vi "Dashboard Main.vi"() -> ()   [LabVIEW 2020]
uses:
  <vilib>/Rock Robotics/WPI/Dashboard/WPI_DashboardLogging Global.vi
  <vilib>/Rock Robotics/Network Tables/NT Read Numeric Array.vi
  <vilib>/Analysis/NI_AALPro.lvlib
  <vilib>/Analysis/coordinate.llb/2D Cartesian Coordinate Rotation (Scalar).vi
  <vilib>/Analysis/NI_AAL_Angle.lvlib
  <vilib>/Analysis/coordinate.llb/Angle Units.ctl
  <vilib>/Analysis/coordinate.llb/Wrap Angle (scalar).vi
panel:
  out "NT Connection":bool
  in  "Camera Settings Right":T1={"Frame Rate"=30, "Compression"=30, "Size"=1, "DB Camera Config"=FALSE} {"Frame Rate" scale=1.0..30.0; "Compression" scale=100.0..-1.0; "Size" items=["640x480", "320x240", "160x120"]}
  in  "Camera Name Right":string(combo)="No Camera Selection"
  out "Camera Perf":string
  in  "Camera Settings":T1={"Frame Rate"=30, "Compression"=30, "Size"=1, "DB Camera Config"=FALSE} {"Frame Rate" scale=1.0..30.0; "Compression" scale=100.0..-1.0; "Size" items=["640x480", "320x240", "160x120"]}
  in  "TCP":refnum<k5>
  in  "Rec Mode":enum32{"Stop", "Record", "Playback"}(radio)
  out "Robot IP":string
  out "Image Message":string="Timeout in Camera Communications"
  in  "Dashboard Tab":T2(tab)
  out "Mode":T3(ring)=enum."Auto Disabled"
  out "Right Camera Perf":cluster{"Bandwidth (Mbps)":dbl, "FPS":dbl}
  out "Swerve Visualizer":cluster{dbl[], dbl[]}[](graph)
  out "Pod Comparisons (Diff -> Setpoint - Actual)":T4
  out "Pose":cluster{"x":dbl, "y":dbl, "theta":dbl}
  out "?":picture
  out "RR":bool=TRUE
  out "Velocity Setpoint":cluster{"vx":dbl, "vy":dbl, "w":dbl}
  out "Estimated Velocity":cluster{"vx":dbl, "vy":dbl, "w":dbl}
  out "Camera Image Right":T5(plugin-control)
  in  "Test Slider":dbl(slide) scale=0.0..100.0 scale format="%#_3g"
  in  "On/Off":bool caption="Solenoid"
  in  "Test Name":u16(ring) items=["Select the test to run..."]
  in  "Test Tree":string(tree)
  in  "Motor":cluster{"Value":dbl, "Enable":bool} {"Value" scale=-1.0..1.0 scale format="%#_3g"}
  out "Progress":T6 {"Test Progress" scale=0.0..100.0}
  in  "Rev/Fwd":cluster{"Forward":bool, "Reverse":bool}
  in  "Test Ring":u16(ring) items=["Monochrome", "Color"]
  out "Tree":string(tree)
  out "Camera Image":T5(plugin-control)
  out "Background":bool
  in  "Camera Name":string(combo)="No Camera Selection"
  # "HW"
  # "HW"
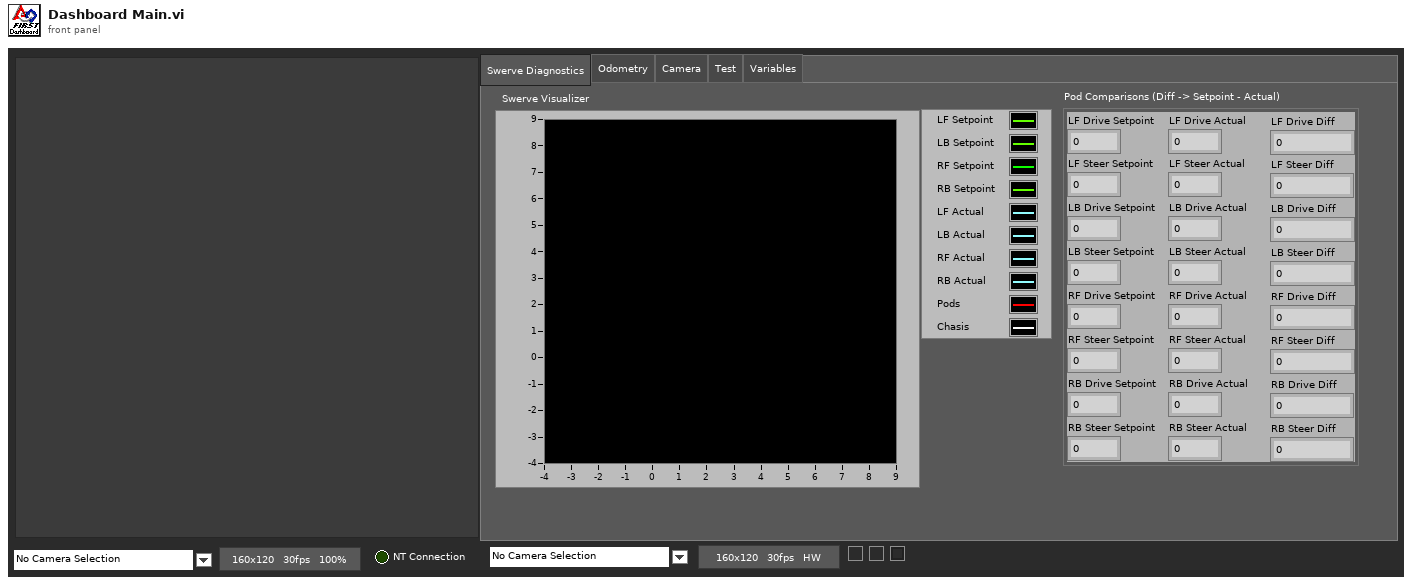
[diagram p1: front panel]
types:
  T1 = cluster{"Frame Rate":i32, "Compression":i32, "Size":u16, "DB Camera Config":bool}
  T2 = enum32{"Swerve Diagnostics", "Odometry", "Camera", "Test", "Variables"}
  T3 = enum8{"Tele-Op Disabled", "Tele-Op Enabled", "Auto Disabled", "Auto Enabled", "Test Disabled", "Test Enabled", "Disconnected", "No Code", "E-Stop"}
  T4 = cluster{"LF Drive Setpoint":dbl, "LF Steer Setpoint":dbl, "LB Drive Setpoint":dbl, "LB Steer Setpoint":dbl, "RF Drive Setpoint":dbl, "RF Steer Setpoint":dbl, "RB Drive Setpoint":dbl, "RB Steer Setpoint":dbl, "LF Drive Actual":dbl, "LF Steer Actual":dbl, "LB Drive Actual":dbl, "LB Steer Actual":dbl, "RF Drive Actual":dbl, "RF Steer Actual":dbl, "RB Drive Actual":dbl, "RB Steer Actual":dbl, "LF Drive Diff":dbl, "LF Steer Diff":dbl, "LB Drive Diff":dbl, "LB Steer Diff":dbl, "RF Drive Diff":dbl, "RF Steer Diff":dbl, "RB Drive Diff":dbl, "RB Steer Diff":dbl}
  T5 = typedef "IMAQ Image.ctl" = refnum<image>
  T6 = cluster{"Test Progress":u8, "Test Progress Text":string}
  T7 = cluster{"Save Path":path, "Interval (s)":dbl, "Keep":i32}
  T8 = typedef "Image Type" = u32
  T9 = cluster{"Error Strings":string, "Disable Counts":cluster{u16, u16}, "Rail Faults":cluster{u16, u16, u16}, "Robot IP":string, "DB Mode":u8, "Event Info":cluster{"Name":string, "Type":u8, "Number":u16, "Replay":u8}}
  T10 = cluster{"Storage":cluster{"Disk Free":u64, "RAM Block":u32, "RAM free":u32}, "CPU Utilization":cluster{"CPU % ISR":sgl, "CPU % Time Crit":sgl, "CPU % Timed Str":sgl, "CPU % High":sgl, "CPU % Above":sgl, "CPU % Normal":sgl, "CPU % Low":sgl}, "CAN":cluster{"% Bus Utilization":sgl, "Bus Off Cnt":u32, "TX_FIFO Full Cnt":u32, "Receive Error Cnt":u8, "Transmit Error Cnt":u8}, "HID":cluster{"HID Outputs":u32, "Rumble Low":u16, "Rumble High":u16}[]}
  T11 = cluster{"Status bits":cluster{"Test Mode":bool, "Autonomous":bool, "Enabled":bool, "Code Start":bool, "Brownout":bool, "Reserved 2":bool, "Reserved 3":bool, "E-Stop":bool}, "Code Trace":cluster{"Disabled":bool, "TeleOp":bool, "Auto":bool, "Test":bool}, "Controller Type":enum16{"unknown", "cRIO", "roboRio"}, "Code?":enum16{"unknown", "noCode", "code"}, "Battery V":dbl}
  T12 = cluster{"Control Bits":cluster{"TestMode":bool, "Autonomous":bool, "Enabled":bool, "FMS Present":bool, bool, bool, bool, "E-Stop":bool}, "Team Station ":u8, "Countdown":sgl, "Joystick Values":cluster{"Axes":dbl[], "Buttons":bool[], "POVs":i16[]}[]}
  T13 = cluster{"value[0]":dbl, "value[1]":dbl, "value[2]":dbl}
  T14 = typedef "NI_AAL_Angle.lvlib/Angle Units.ctl" = i32
  T15 = cluster{"[0]":dbl, "[1]":dbl, "[2]":dbl, "[3]":dbl, "[4]":dbl, "[5]":dbl, "[6]":dbl, "[7]":dbl, "[8]":dbl, "[9]":dbl, "[10]":dbl, "[11]":dbl, "[12]":dbl, "[13]":dbl, "[14]":dbl, "[15]":dbl, "[16]":dbl, "[17]":dbl, "[18]":dbl, "[19]":dbl, "[20]":dbl, "[21]":dbl, "[22]":dbl, "[23]":dbl}
  T16 = typedef "LVPositionTypeDef.ctl" = cluster{"Left":i32, "Top":i32}
  T17 = typedef "LVBoundsTypeDef.ctl" = cluster{"Width":u32, "Height":u32}
  T18 = cluster{"Global Rectangle":i32[], "Contours":cluster{"Contour Type":u32, "ROI Type":u32, "Points":i32[]}[]}
  T19 = cluster{"Camera Name":string, string, "Saved DB Images Info":cluster{"Save Path":path, "Interval (s)":dbl, "Keep":i32}}
  T20 = cluster{"Camera Name Right":string, string, "Saved DB Images Info":cluster{"Save Path":path, "Interval (s)":dbl, "Keep":i32}}
  T21 = cluster{"x out":dbl, "y out":dbl, "value[2]":dbl}
  T22 = typedef "LVPoint32TypeDef.ctl" = cluster{"Horizontal":i32, "Vertical":i32}
  T23 = cluster{"Operation":enum16{"Update", "Clear"}, "Color Box":u32}[]
  T24 = cluster{"Image Size":bool, "Image Type":bool, "Pixel Value":bool, "ROI Information":bool, "Zoom Factor":bool}
  T25 = cluster{"Operation":enum16{"Update", "Clear"}, "Color Box":u32}
  T26 = cluster{"Shift":bool, "Ctrl":bool, "Alt":bool, "Cmd":bool, "Opt":bool}
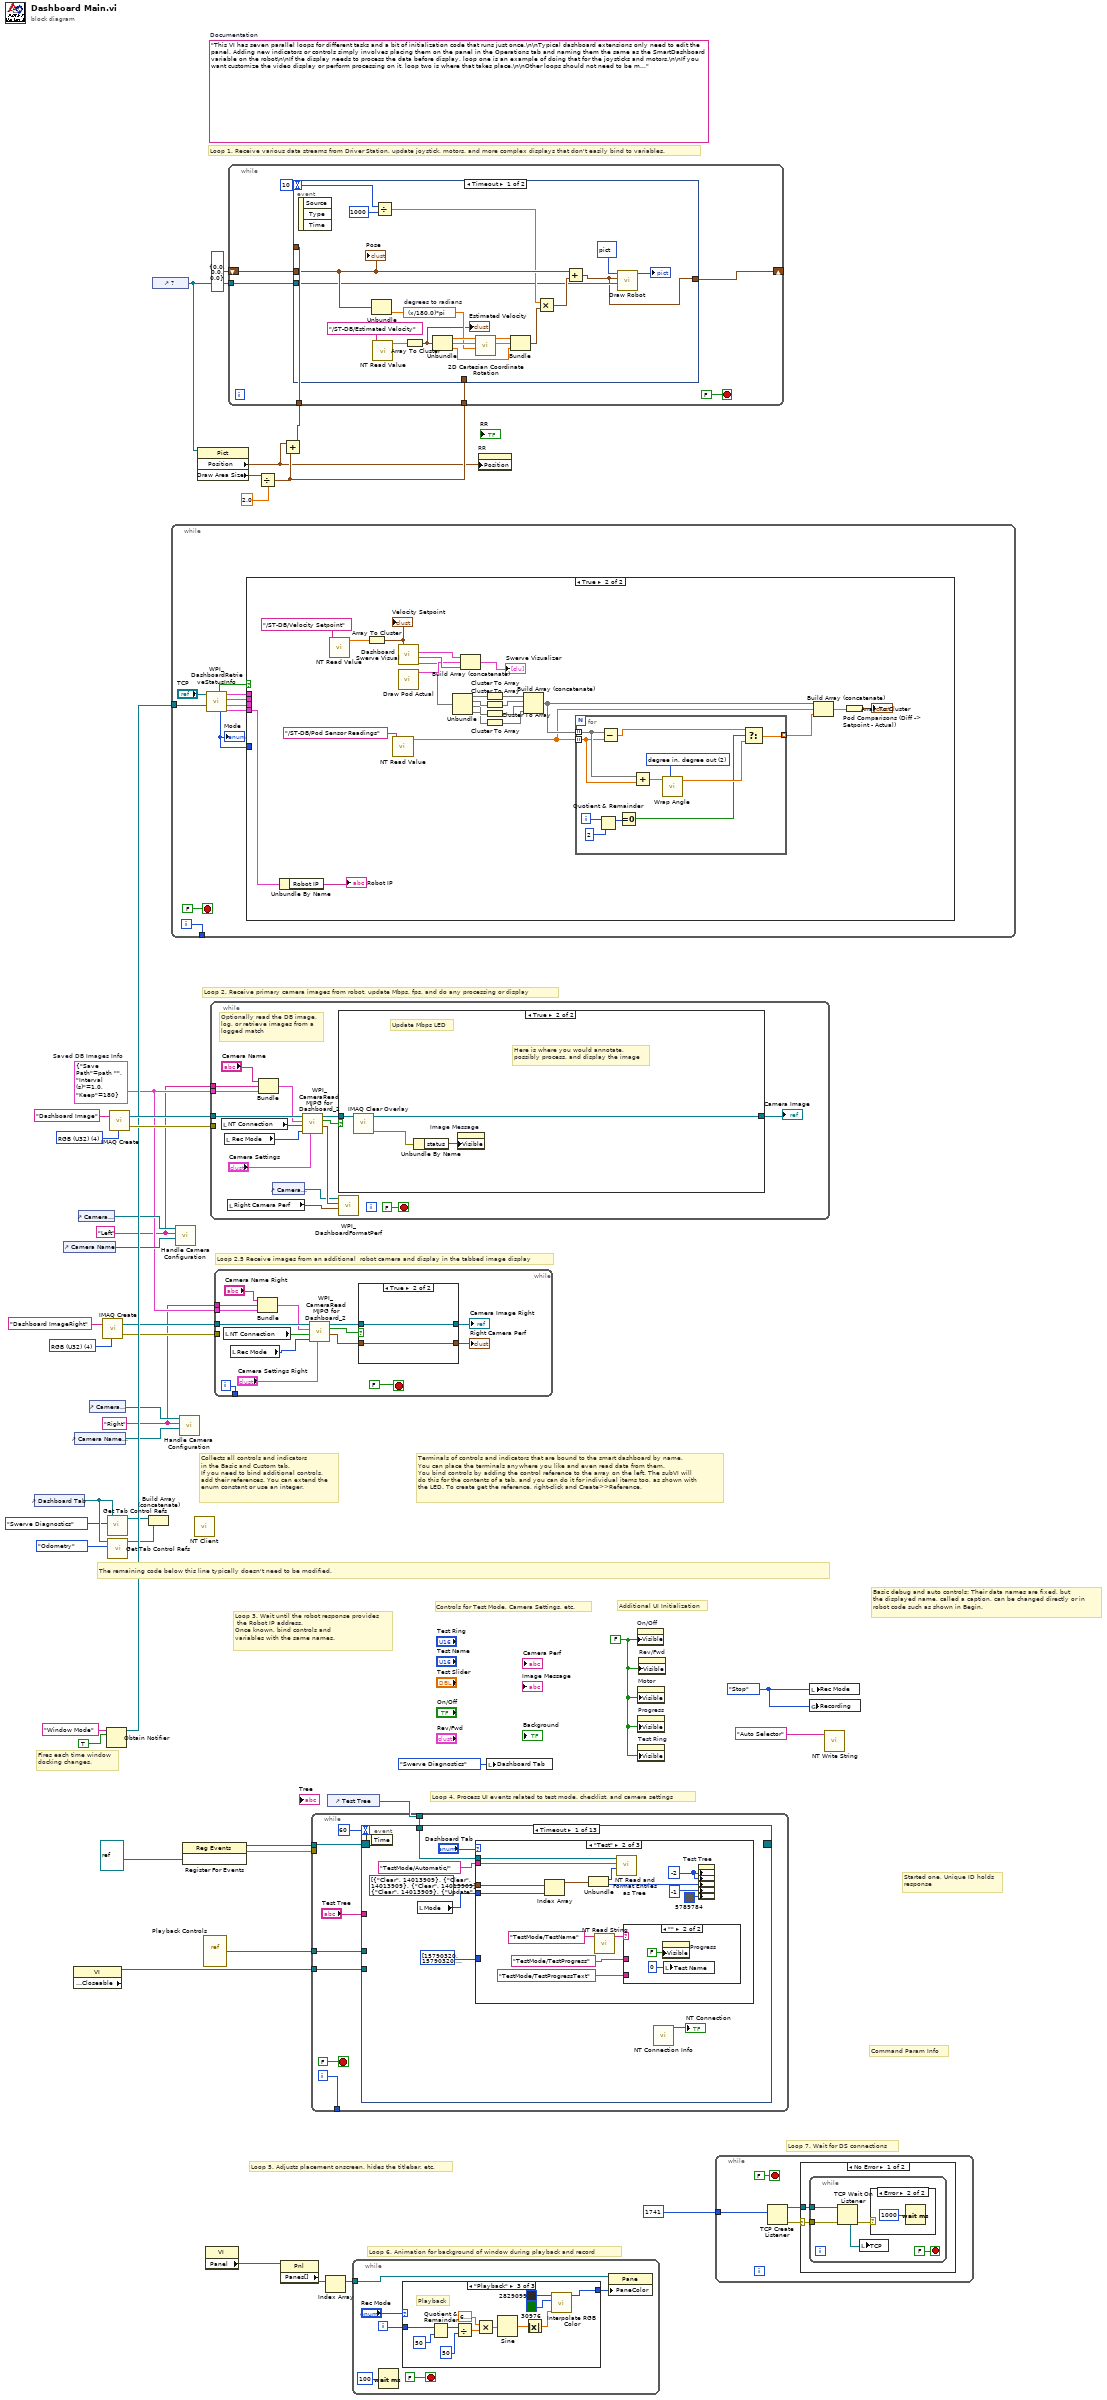
[diagram p0: block diagram]
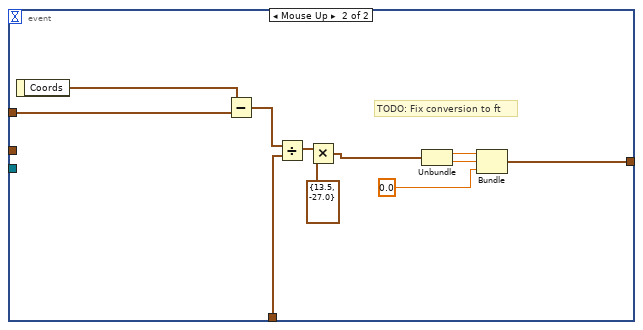
[diagram p2: hidden frame]
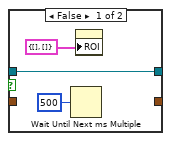
[diagram p3: hidden frame]
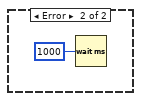
[diagram p5: hidden frame]
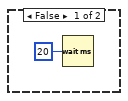
[diagram p6: hidden frame]
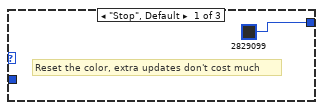
[diagram p7: hidden frame]
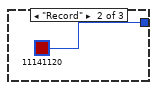
[diagram p8: hidden frame]
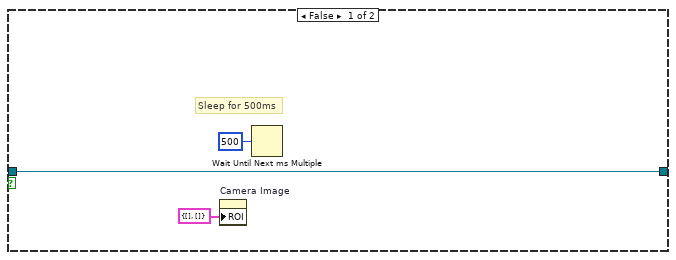
[diagram p9: hidden frame]
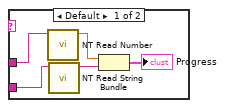
[diagram p11: hidden frame]
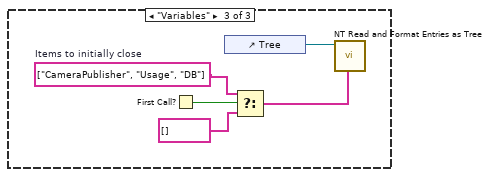
[diagram p12: hidden frame]
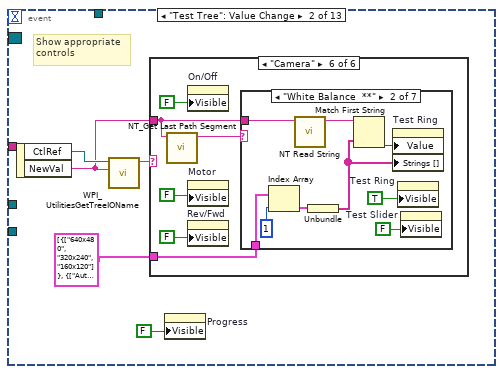
[diagram p13: hidden frame]
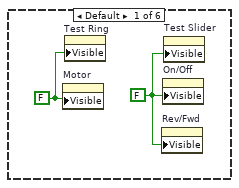
[diagram p14: hidden frame]
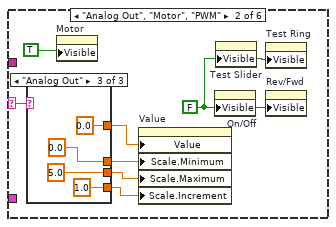
[diagram p15: hidden frame]
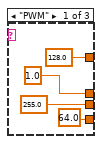
[diagram p16: hidden frame]
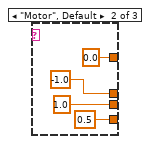
[diagram p17: hidden frame]
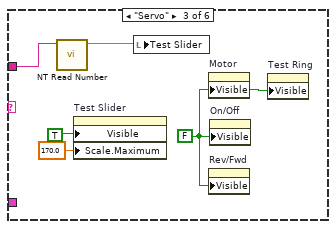
[diagram p18: hidden frame]
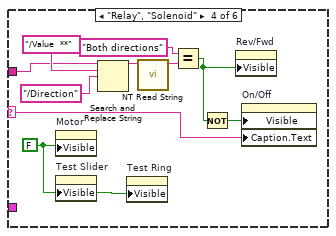
[diagram p19: hidden frame]
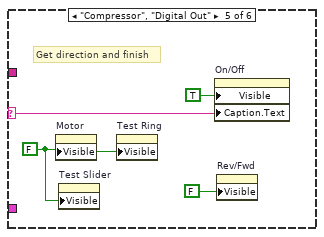
[diagram p20: hidden frame]
diagram:
  w16 = T7 {"Save Path"=path "", "Interval (s)"=1.0, "Keep"=180}  # Saved DB Images Info
  w15 = "Right"
  w14 = "Left"
  w21 = T8 4 items=["Grayscale (U8)", "Grayscale (I16)", "Grayscale (SGL)", "Complex (CSG)", "RGB (U32)", "HSL (U32)", "RGB (U64)"] ("Image Type")
  w30 = enum32{"Stop", "Record", "Playback"}."Stop" ("Rec Mode")
  w28 = FALSE ("Visible")
  (unwired) "This VI has seven parallel loops for different tasks and a bit of initialization code that runs just once.\n\nTypical dashboard extensions only need to edit the panel. Adding new indicators or controls simply involves placing them on the panel in the Operations tab and naming them the same as the SmartDashboard variable on the robot\n\nIf the display needs to process the data before display, loop one is an example of doing that for the joysticks and motors.\n\nIf you want customize the video display or perform processing on it, loop two is where that takes place.\n\nOther loops should not need to be modified. They are pretty standard, and document the task they perform."  # Documentation
  w44 = T8 4 items=["Grayscale (U8)", "Grayscale (I16)", "Grayscale (SGL)", "Complex (CSG)", "RGB (U32)", "HSL (U32)", "RGB (U64)"] ("Image Type")
  # "Collects all controls and indicators\nin the Basic and Custom tab.\nIf you need to bind additional controls,\nadd their references. You can extend the\nenum constant or use an integer."
  # "Loop 2.5 Receive images from an additional  robot camera and display in the tabbed image display"
  # "Command Param Info"
  # "Started one, Unique ID holds\nresponse"
  # "Loop 7. Wait for DS connections"
  # "Basic debug and auto controls: Their data names are fixed, but\nthe displayed name, called a caption, can be changed directly or in\nrobot code such as shown in Begin."
  # "Controls for Test Mode, Camera Settings, etc."
  # "Additional UI Initialization"
  # "Loop 6. Animation for background of window during playback and record"
  # "Fires each time window\ndocking changes."
  # "The remaining code below this line typically doesn't need to be modified."
  # "Loop 4. Process UI events related to test mode, checklist, and camera settings"
  # "Terminals of controls and indicators that are bound to the smart dashboard by name.\nYou can place the terminals anywhere you like and even read data from them.\nYou bind controls by adding the control reference to the array on the left. The subVI will\ndo this for the contents of a tab, and you can do it for individual items too, as shown with\nthe LED. To create get the reference, right-click and Create>>Reference."
  # "Loop 3. Wait until the robot response provides\n the Robot IP address.\nOnce known, bind controls and\nvariables with the same names."
  # "Loop 5. Adjusts placement onscreen, hides the titlebar, etc."
  # "Loop 1. Receive various data streams from Driver Station, update joystick, motors, and more complex displays that don't easily bind to variables."
  # "Loop 2. Receive primary camera images from robot, update Mbps, fps, and do any processing or display"
  n1 = control-ref of="Dashboard Tab"() -> (w5:refnum<vi>)
  n2 = control-ref of="Camera Name"() -> (w24:refnum<vi>)
  n3 = property class="VI" props=["Front Panel.Closeable"]() -> (reference out=w29:refnum<vi>)  [unwired: 2 in, 2 out]
  n4 = control-ref of="Camera Name Right"() -> (w17:refnum<vi>)
  n5 = control-ref of="Camera Settings"() -> (w25:refnum<vi>)
  n6 = control-ref of="Camera Settings Right"() -> (w18:refnum<vi>)
  n7 = call "IMAQ Create"("Image Name"="Dashboard ImageRight", "Image Type"=w21) -> ("New Image"=w20:T5, "error out"=w19:errorcluster)  [unwired: 2 in, 1 out]
  n8 = Obtain Notifier(name (unnamed)="Window Mode", notification data type=TRUE) -> (notifier out=w27:refnum<notifier>)  [unwired: 2 in, 2 out]
  n9 = call <vilib>:"Get Tab Control Refs.vi"("Page Index"=T2."Swerve Diagnostics" ("Dashboard Tab"), "TabControl in"=w5) -> ("ControlsOnPage"=w4:refnum<vi>[])  [unwired: 9 in]
  n10 = call <vilib>:"Get Tab Control Refs.vi"("Page Index"=T2."Odometry" ("Dashboard Tab"), "TabControl in"=w5) -> ("ControlsOnPage"=w3:refnum<vi>[])  [unwired: 9 in]
  n11 = call "IMAQ Create"("Image Name"="Dashboard Image", "Image Type"=w44) -> ("New Image"=w42:T5, "error out"=w41:errorcluster)  [unwired: 2 in, 1 out]
  n12 = Build Array (concatenate)(w4, w3) -> ()  [unwired: 1 out]
  n13 = control-ref of="?"() -> (w12:refnum<vi>)
  n14 = while {
    tunnel: [w53] -> _
    tunnel: w27 -> [w45]
    i -> [w53]
    stop <- FALSE stop-if-true
    n15 = call <vilib>:"WPI_DashboardRetrieveStatusInfo.vi"("Window Mode Notifier"=w45, "TCP Cnx"="TCP") -> ("Power and Errors"=w48:T9, "Robot Metrics"=w51:T10, "Status Info"=w52:T11, "Control Info"=w49:T12, "Robot Mode"=w47:T3, "Process?"=w50:bool)  [unwired: 4 in]
    "Mode" <- w47
    n16 = case shown="True" w50 {
      tunnel: w52 -> [_ _]
      tunnel: w51 -> [_ _]
      tunnel: w49 -> [_ _]
      tunnel: w48 -> [_ w79]
      tunnel: w47 -> [_ _]
      frame False {
        n17 = Wait (ms)(milliseconds to wait=u32 20) -> ()  [unwired: 1 out]
      }
      frame True {
        n18 = Unbundle By Name(w79) -> ("Robot IP"=→"Robot IP":string)
        n19 = call-poly <vilib>:"NT Read Value.vi"("name"="/ST-DB/Velocity Setpoint") -> ("value"=w72:dbl[])  [unwired: 8 in, 2 out]
        n20 = Array To Cluster(array=w72) -> (cluster=w71:T13)
        "Velocity Setpoint" <- w71
        n21 = call-poly <vilib>:"NT Read Value.vi"("name"="/ST-DB/Pod Sensor Readings") -> ("value"=w56:dbl[])  [unwired: 8 in, 2 out]
        n22 = call "Dashboard Swerve Visual.vi"(11:w71) -> (0:w69, 1:w76, "Robot"=w74:cluster{dbl[], dbl[]}[])  [unwired: 7 in, 1 out]
        n23 = call "Draw Pod Actual.vi"() -> ("Actual Pod Vectors"=w75:cluster{dbl[], dbl[]}[])  [unwired: 11 in]
        n24 = Unbundle(w69) -> ("Left Front"=w68, "Left Back"=w67, "Right Front"=w66, "Right Back"=w65)
        n25 = Build Array (concatenate)(w74, w75, w76) -> (→"Swerve Visualizer":cluster{dbl[], dbl[]}[])
        n26 = Cluster To Array(cluster=w68) -> (array=w64:void[])
        n27 = Cluster To Array(cluster=w67) -> (array=w63:void[])
        n28 = Cluster To Array(cluster=w66) -> (array=w62:void[])
        n29 = Cluster To Array(cluster=w65) -> (array=w61:void[])
        n30 = Build Array (concatenate)(w64, w63, w62, w61) -> (w57:void[])
        n31 = for {
          tunnel: [w83] -> w58 mode=indexing
          tunnel: w57 -> [w82] mode=indexing
          tunnel: w56 -> [w81] mode=indexing
          i -> [w90]
          w86 = T14 2 items=["radian in, radian out", "radian in, degree out", "degree in, degree out", "degree in, radian out"] ("angle units")
          n32 = Quotient & Remainder(x=w90, y=2) -> (x-y*floor(x/y)=w88:i32)  [unwired: 1 out]
          n33 = Subtract(x=w82, y=w81) -> (x-y=w80:dbl)
          n34 = Equal To 0?(x=w88) -> (x = 0?=w84:bool)
          n35 = Add(x=w82, y=w81) -> (x+y=w87:dbl)
          n36 = call-poly <vilib>:"Wrap Angle.vi"("angle units"=w86, "angle in"=w87) -> ("angle out"=w85:dbl)  [unwired: 8 in, 1 out]
          n37 = Select(t=w80, s=w84, f=w85) -> (s? t:f=w83:dbl)
        }
        n38 = Build Array (concatenate)(w57, w56, w58) -> (w60:dbl[])
        n39 = Array To Cluster(array=w60) -> (cluster=→"Pod Comparisons (Diff -> Setpoint - Actual)":T15)
      }
    }
  }
  n40 = call "Handle Camera Configuration.vi"("CameraNameRef"=w24, "Display Name"=w14, "ClusterRef"=w25) -> ()  [unwired: 9 in]
  n41 = call "Handle Camera Configuration.vi"("CameraNameRef"=w17, "Display Name"=w15, "ClusterRef"=w18) -> ()  [unwired: 9 in]
  n42 = register-events(refnum<vi> refnum) -> (reference out=w33:refnum<event-registration>, error out=w32:errorcluster)  [unwired: 2 in]
  n43 = call <vilib>:"NT Client.vi"() -> ()  [unwired: 11 in, 1 out]
  n44 = property class="Pict"(reference=w12) -> ("Position"=w7:T16, "Draw Area Size"=w11:T17)  [unwired: 1 in, 2 out]
  n45 = vi-ref "Playback Controls.vi"() -> (w34:refnum<vi>)
  n46 = property class="VI"() -> ("Panel"=w36:refnum<vi>)  [unwired: 2 in, 2 out]
  n47 = while {
    tunnel: w42 -> [w104]
    tunnel: w41 -> [_]
    tunnel: w16 -> [w97]
    tunnel: w14 -> [w94]
    stop <- FALSE stop-if-true
    # "Optionally read the DB image,\nlog, or retrieve images from a\nlogged match"
    n48 = local read "NT Connection"() -> (w98:bool)
    n49 = local read "Rec Mode"() -> (w101:enum32{"Stop", "Record", "Playback"})
    n50 = local read "Right Camera Perf"() -> (w92:cluster{"Bandwidth (Mbps)":dbl, "FPS":dbl})
    n51 = Bundle("Camera Name"="Camera Name", w94, "Saved DB Images Info"=w97) -> (w96:T19)  [unwired: 1 in]
    n52 = control-ref of="Camera Perf"() -> (w91:refnum<vi>)
    n53 = call <vilib>:"WPI_CameraRead MJPG for Dashboard_2.vi"("Camera Settings"="Camera Settings", "Rec Mode"=w101, "NT Connection"=w98, "Capture Info"=w96, "Image in"=w104) -> ("perf info"=w93:cluster{"Bandwidth (Mbps)":dbl, "fps":dbl}, "Active"=w102:bool, "Image\\ out"=w103:T5)  [unwired: 4 in]
    n54 = case shown="True" w102 {
      tunnel: w103 -> [w107 w110]
      tunnel: [w107 w109] -> w99
      frame False {
        # "Sleep for 500ms"
        n55 = property on="Camera Image" class="ImageControl"("ROI"=T18 {"Global Rectangle"=[], "Contours"=[]}) -> ()  [unwired: 2 in, 2 out]
        n56 = Wait Until Next ms Multiple(millisecond multiple=u32 500) -> ()  [unwired: 1 out]
      }
      frame True {
        # "Here is where you would annotate,\npossibly process, and display the image"
        # "Update Mbps LED"
        n57 = call "IMAQ Clear Overlay"("Image"=w110) -> ("error out"=w111:errorcluster, "Image Out"=w109:T5)  [unwired: 2 in, 7 out]
        n58 = Unbundle By Name(w111) -> ("status"=w112:bool)
        n59 = property on="Image Message" class="Str"("Visible"=w112) -> ()  [unwired: 2 in, 2 out]
      }
    }
    "Camera Image" <- w99
    n60 = call <vilib>:"WPI_DashboardFormatPerf.vi"("Right Camera Perf"=w92, "Performance"=w93, "String in"=w91) -> ()  [unwired: 9 in]
  }
  n61 = while {
    tunnel: w20 -> [w127]
    tunnel: w19 -> [_]
    tunnel: [w122] -> _
    tunnel: w16 -> [w118]
    tunnel: w15 -> [w115]
    i -> [w122]
    stop <- FALSE stop-if-true
    n62 = local read "NT Connection"() -> (w119:bool)
    n63 = local read "Rec Mode"() -> (w126:enum32{"Stop", "Record", "Playback"})
    n64 = Bundle("Camera Name Right"="Camera Name Right", w115, "Saved DB Images Info"=w118) -> (w117:T20)  [unwired: 1 in]
    n65 = call <vilib>:"WPI_CameraRead MJPG for Dashboard_2.vi"("Camera Settings"="Camera Settings Right", "Rec Mode"=w126, "NT Connection"=w119, "Capture Info"=w117, "Image in"=w127) -> ("perf info"=w113:cluster{"Bandwidth (Mbps)":dbl, "fps":dbl}, "Active"=w121:bool, "Image\\ out"=w124:T5)  [unwired: 4 in]
    n66 = case shown="True" w121 {
      tunnel: w124 -> [w129 w132]
      tunnel: [w129 w132] -> w120
      tunnel: [_ w131] -> w114
      tunnel: w113 -> [_ w131]
      frame False {
        n67 = Wait Until Next ms Multiple(millisecond multiple=u32 500) -> ()  [unwired: 1 out]
        n68 = property on="Camera Image Right" class="ImageControl"("ROI"=T18 {"Global Rectangle"=[], "Contours"=[]}) -> ()  [unwired: 2 in, 2 out]
      }
      frame True {
      }
    }
    "Camera Image Right" <- w120
    "Right Camera Perf" <- w114
  }
  n69 = Divide(x=w11, y=2.0) -> (x/y=w8:cluster{"Width":dbl, "Height":dbl})
  n70 = property class="Pnl"(reference=w36) -> ("Panes[]"=w37:refnum<vi>[])  [unwired: 1 in, 2 out]
  n71 = Add(x=w7, y=w8) -> (x+y=w9:cluster{dbl, dbl})
  n72 = while {
    tunnel: w12 -> [w137]
    tunnel: w9 -> [w136]
    tunnel: w8 -> [w135]
    shift-right: [w134] -> _
    shift-left: cluster{dbl, dbl, dbl} {0.0, 0.0, 0.0} -> [w133]
    stop <- FALSE stop-if-true
    n73 = event shown="[0] Timeout" {
      selector: _ -> [_ _]
      dyn-events: _ -> [_ _]
      timeout: 10 -> [w158 _]
      tunnel: w137 -> [w144 _]
      tunnel: w136 -> [_ w170]
      tunnel: w135 -> [_ w164]
      tunnel: [w143 w160] -> w134
      tunnel: w133 -> [w149 _]
      event Timeout {
        n74 = event-data() -> ()  [unwired: 1 in, 3 out]
        n75 = Unbundle(w149) -> (w148:dbl)  [unwired: 2 out]
        n76 = call-poly <vilib>:"NT Read Value.vi"("name"="/ST-DB/Estimated Velocity") -> ("value"=w141:dbl[])  [unwired: 8 in, 2 out]
        n77 = Divide(x=w158, y=1000) -> (x/y=w147:dbl)
        n78 = expression code="(x/180.0)*pi" "degrees to radians"(w148) -> (w150:dbl)
        n79 = Array To Cluster(array=w141) -> (cluster=w142:T13)
        "Estimated Velocity" <- w142
        n80 = Unbundle(w142) -> ("value[0]"=w156:dbl, "value[1]"=w155:dbl, "value[2]"=w152:dbl)
        n81 = call-poly <vilib>:"2D Cartesian Coordinate Rotation.vi"("theta"=w150, "y"=w155, "x"=w156) -> ("y out"=w153:dbl, "x out"=w154:dbl)  [unwired: 6 in, 1 out]
        n82 = Bundle("x out"=w154, "y out"=w153, "value[2]"=w152) -> (w151:T21)  [unwired: 1 in]
        n83 = Multiply(x=w147, y=w151) -> (x*y=w159:T21)
        n84 = Add(x=w149, y=w159) -> (x+y=w143:cluster{dbl, dbl, dbl})
        n85 = call "Draw Robot.vi"("Picture  Reference"=w144, "Pose"=w143, "Picture In"=picture data[5B]) -> ("Picture Out"=→"?":picture)  [unwired: 8 in]
        "Pose" <- w149
      }
      event Mouse Up {
        # "TODO: Fix conversion to ft"
        n86 = event-data() -> ("Coords"=w169:T22)  [unwired: 1 in]
        n87 = Subtract(x=w169, y=w170) -> (x-y=w165:cluster{dbl, dbl})
        n88 = Divide(x=w165, y=w164) -> (x/y=w163:cluster{dbl, dbl})
        n89 = Multiply(x=w163, y=cluster{dbl, dbl} {13.5, -27.0}) -> (x*y=w161:cluster{dbl, dbl})
        n90 = Unbundle(w161) -> (w168:dbl, w167:dbl)
        n91 = Bundle(w168, w167, 0.0) -> (w160:cluster{dbl, dbl, dbl})  [unwired: 1 in]
      }
    }
  }
  n92 = Index Array(array=w37) -> (element=w35:refnum<vi>)  [unwired: 1 in]
  n93 = control-ref of="Test Tree"() -> (w38:refnum<vi>)
  n94 = while {
    tunnel: [w175] -> _
    tunnel: w38 -> [w174]
    tunnel: w34 -> [w173]
    tunnel: w33 -> [w172]
    tunnel: w32 -> [_]
    tunnel: w29 -> [w171]
    i -> [w175]
    stop <- FALSE stop-if-true
    n95 = event shown="[0] Timeout" {
      selector: w172 -> [_ _ _ _ _ _ _ _ _ _ _ _ _]
      dyn-events: [_ _ _ _ _ _ _ _ _ w352 _ _ _] -> _
      timeout: u32 60 ("milliseconds to wait") -> [_ _ _ _ _ _ _ _ _ _ _ _ _]
      tunnel: w174 -> [w184 _ _ _ _ _ _ _ _ _ _ _ _]
      tunnel: "Test Tree" -> [_ _ _ _ w325 w332 w333 w336 w343 _ _ _ _]
      tunnel: w173 -> [_ _ _ _ _ _ _ _ _ w354 _ w369 _]
      tunnel: w171 -> [_ _ _ _ _ _ _ _ _ w350 _ _ _]
      event Timeout {
        n96 = event-data() -> ()  [unwired: 1 in, 1 out]
        n97 = local read "Mode"() -> (w182:T3)
        n98 = case shown="\"Test\"" "Dashboard Tab" {
          tunnel: w184 -> [_ w199 _]
          tunnel: "TestMode/Automatic/" ("Name Pattern") -> [_ w198 _]
          tunnel: T23 [{"Operation"=enum."Clear", "Color Box"=14013909}, {"Operation"=enum."Clear", "Color Box"=14013909}, {"Operation"=enum."Clear", "Color Box"=14013909}, {"Operation"=enum."Clear", "Color Box"=14013909}, {"Operation"=enum."Update", "Color Box"=14013909}, {"Operation"=enum."Update", "Color Box"=16777215}, {"Operation"=enum."Clear", "Color Box"=14013909}, {"Operation"=enum."Clear", "Color Box"=14013909}, {"Operation"=enum."Clear", "Color Box"=14013909}] -> [_ w191 _]
          tunnel: w182 -> [_ w190 _]
          tunnel: u32[] [15790320, 15790320, 15790320, 15790320, 16777215, 16777215, 15790320, 15790320, 15790320] -> [_ _ _]
          frame Default {
          }
          frame "Test" {
            w197 = -2 ("Active Item:Row Number")
            n99 = Index Array(array=w191, index=w190) -> (element=w192:T25)
            n100 = Unbundle(w192) -> ("Operation"=w193:enum16{"Update", "Clear"}, "Color Box"=w194:u32)
            n101 = call <vilib>:"NT Read String.vi"("name"="TestMode/TestName" ("Name")) -> ("value"=w188:string)  [unwired: 8 in, 2 out]
            n102 = call <vilib>:"NT Read and Format Entries as Tree.vi"("Operation"=w193, "Name Pattern"=w198, "Tree Refnum"=w199) -> ()  [unwired: 7 in, 2 out]
            n103 = case shown="\"\"" w188 {
              tunnel: "TestMode/TestProgress" ("Name") -> [w201 _]
              tunnel: "TestMode/TestProgressText" ("Name") -> [w200 _]
              frame Default {
                n104 = call <vilib>:"NT Read Number.vi"("name"=w201) -> ("value"=w202:dbl)  [unwired: 8 in, 2 out]
                n105 = call <vilib>:"NT Read String.vi"("name"=w200) -> ("value"=w203:string)  [unwired: 8 in, 2 out]
                n106 = Bundle("value"=w202, "value"=w203) -> (→"Progress":cluster{"value":dbl, "value":string})  [unwired: 1 in]
              }
              frame "" {
                n107 = property on="Progress" class="Clust (strict)"("Visible"=FALSE) -> ()  [unwired: 2 in, 2 out]
                n108 = local write "Test Name"(u16 0) -> ()
              }
            }
            n109 = property on="Test Tree" class="Tree (strict)"("Active Item Row Number"=w197, "ActiveColNum"=w197, "CellBG"=w194, "Active Item Row Number"=-1 ("Active Item:Row Number"), "CellBG"=u32 5789784 ("Color Box")) -> ()  [unwired: 2 in, 2 out]
          }
          frame "Variables" {
            w209 = string[] ["CameraPublisher", "Usage", "DB"]  # Items to initially close
            n110 = First Call?() -> (First Call?: T/F=w210:bool)
            n111 = control-ref of="Tree"() -> (w211:refnum<vi>)
            n112 = Select(t=w209, s=w210, f=string[] []) -> (s? t:f=w207:string[])
            n113 = call <vilib>:"NT Read and Format Entries as Tree.vi"("Tags to  Close"=w207, "Tree Refnum"=w211) -> ()  [unwired: 8 in, 2 out]
          }
        }
        n114 = call <vilib>:"NT Connection Info.vi"() -> ("Connected"=→"NT Connection":bool)  [unwired: 11 in]
      }
      event "Test Tree": Value Change {
        # "Show appropriate\ncontrols"
        n115 = event-data() -> ("CtlRef"=w215:refnum<vi>, "NewVal"=w213:string)  [unwired: 1 in]
        n116 = call <vilib>:"WPI_UtilitiesGetTreeIOName.vi"("NewVal"=w213, "TreeControl in"=w215) -> ("I/O Name"=w216:string)  [unwired: 9 in]
        n117 = case shown="\"Camera\"" w216 {
          selector: w216 -> [_ w223 _ w245 w254 _]
          tunnel: w213 -> [_ _ w242 w244 _ w261]
          tunnel: cluster{string[]}[] [{["640x480", "320x240", "160x120"]}, {["Auto", "Fixed indoor", "Fixed outdoor 1", "Fixed outdoor 2", "Fixed fluorescent 1", "Fixed fluorescent 2", "Hold current"]}, {["Auto", "Flicker-free 50 Hz", "Flicker-free 60 Hz", "Hold current"]}, {["None", "Prioritize frame rate", "Prioritize image quality"]}, {["Monochrome", "Color"]}] -> [_ _ _ _ _ w260]
          frame Default {
            w218 = FALSE ("Visible")
            w217 = FALSE ("Visible")
            n118 = property on="Motor" class="Clust (strict)"("Visible"=w217) -> ()  [unwired: 2 in, 2 out]
            n119 = property on="Test Ring" class="Ring (strict)"("Visible"=w217) -> ()  [unwired: 2 in, 2 out]
            n120 = property on="Rev/Fwd" class="Clust (strict)"("Visible"=w218) -> ()  [unwired: 2 in, 2 out]
            n121 = property on="On/Off" class="Bool (strict)"("Visible"=w218) -> ()  [unwired: 2 in, 2 out]
            n122 = property on="Test Slider" class="Slide (strict)"("Visible"=w218) -> ()  [unwired: 2 in, 2 out]
          }
          frame "Analog Out", "Motor", "PWM" {
            w224 = FALSE ("Visible")
            n123 = case shown="\"Analog Out\"" w223 {
              tunnel: [1.0 ("Value") -1.0 ("Value") 0.0 ("Value")] -> w222
              tunnel: [255.0 ("Value") 1.0 ("Value") 5.0 ("Value")] -> w221
              tunnel: [128.0 ("Value") 0.0 ("Value") 0.0 ("Value")] -> w220
              tunnel: [64.0 ("Value") 0.5 ("Value") 1.0 ("Value")] -> w219
              frame "PWM" {
              }
              frame "Motor", Default {
              }
              frame "Analog Out" {
              }
            }
            n124 = property on="Motor" class="Clust (strict)"("Visible"=TRUE) -> ()  [unwired: 2 in, 2 out]
            n125 = property on="Value" class="Slide (strict)"("Value"=w220, "Scale.Minimum"=w222, "Scale.Maximum"=w221, "Scale.Increment"=w219) -> ()  [unwired: 2 in, 2 out]
            n126 = property on="On/Off" class="Bool (strict)"("Visible"=w224) -> ()  [unwired: 2 in, 2 out]
            n127 = property on="Test Slider" class="Slide (strict)"("Visible"=w224) -> ()  [unwired: 2 in, 2 out]
            n128 = property on="Test Ring" class="Ring (strict)"("Visible"=w224) -> ()  [unwired: 2 in, 2 out]
            n129 = property on="Rev/Fwd" class="Clust (strict)"("Visible"=w224) -> ()  [unwired: 2 in, 2 out]
          }
          frame "Servo" {
            w240 = FALSE ("Visible")
            n130 = call <vilib>:"NT Read Number.vi"("name"=w242) -> ("value"=w241:dbl)  [unwired: 8 in, 2 out]
            n131 = property on="Test Slider" class="Slide (strict)"("Visible"=TRUE, "Scale.Maximum"=170.0 ("Scale.Range:Maximum")) -> ()  [unwired: 2 in, 2 out]
            n132 = local write "Test Slider"(w241) -> ()
            n133 = property on="Motor" class="Clust (strict)"("Visible"=w240) -> ()  [unwired: 2 in, 2 out]
            n134 = property on="Rev/Fwd" class="Clust (strict)"("Visible"=w240) -> ()  [unwired: 2 in, 2 out]
            n135 = property on="On/Off" class="Bool (strict)"("Visible"=w240) -> ()  [unwired: 2 in, 2 out]
            n136 = property on="Test Ring" class="Ring (strict)"("Visible"=w240) -> ()  [unwired: 2 in, 2 out]
          }
          frame "Relay", "Solenoid" {
            w243 = FALSE ("Visible")
            n137 = property on="Motor" class="Clust (strict)"("Visible"=w243) -> ()  [unwired: 2 in, 2 out]
            n138 = property on="Test Slider" class="Slide (strict)"("Visible"=w243) -> ()  [unwired: 2 in, 2 out]
            n139 = Search and Replace String(input string=w244, search string="/Value  **", replace string="/Direction") -> (result string=w250:string)  [unwired: 5 in, 3 out]
            n140 = property on="Test Ring" class="Ring (strict)"("Visible"=w243) -> ()  [unwired: 2 in, 2 out]
            n141 = call <vilib>:"NT Read String.vi"("name"=w250) -> ("value"=w248:string)  [unwired: 8 in, 2 out]
            n142 = Equal?(x="Both directions", y=w248) -> (x = y?=w246:bool)
            n143 = Not(x=w246) -> (.not. x?=w247:bool)
            n144 = property on="Rev/Fwd" class="Clust (strict)"("Visible"=w246) -> ()  [unwired: 2 in, 2 out]
            n145 = property on="On/Off" class="Bool (strict)"("Visible"=w247, "Caption.Text"=w245) -> ()  [unwired: 2 in, 2 out]
          }
          frame "Compressor", "Digital Out" {
            w253 = FALSE ("Visible")
            # "Get direction and finish"
            n146 = property on="Motor" class="Clust (strict)"("Visible"=w253) -> ()  [unwired: 2 in, 2 out]
            n147 = property on="Test Slider" class="Slide (strict)"("Visible"=w253) -> ()  [unwired: 2 in, 2 out]
            n148 = property on="Test Ring" class="Ring (strict)"("Visible"=w253) -> ()  [unwired: 2 in, 2 out]
            n149 = property on="On/Off" class="Bool (strict)"("Visible"=TRUE, "Caption.Text"=w254) -> ()  [unwired: 2 in, 2 out]
            n150 = property on="Rev/Fwd" class="Clust (strict)"("Visible"=FALSE) -> ()  [unwired: 2 in, 2 out]
          }
          frame "Camera" {
            n151 = call <vilib>:"NT_Get Last Path Segment.vi"("String in"=w261) -> ("String out"=w262:string)  [unwired: 10 in]
            n152 = property on="On/Off" class="Bool (strict)"("Visible"=FALSE) -> ()  [unwired: 2 in, 2 out]
            n153 = property on="Motor" class="Clust (strict)"("Visible"=FALSE) -> ()  [unwired: 2 in, 2 out]
            n154 = property on="Rev/Fwd" class="Clust (strict)"("Visible"=FALSE) -> ()  [unwired: 2 in, 2 out]
            n155 = case shown="\"White Balance  **\"" w262 {
              tunnel: w261 -> [w268 w277 w286 w295 w304 _ w310]
              tunnel: w260 -> [w266 w274 w283 w292 w301 _ _]
              frame "Size  **" {
                n156 = Index Array(array=w266) -> (element=w265:cluster{string[]})  [unwired: 1 in]
                n157 = call <vilib>:"NT Read String.vi"("name"=w268) -> ("value"=w267:string)  [unwired: 8 in, 2 out]
                n158 = Unbundle(w265) -> (w263:string[])
                n159 = Match First String(2:w263, 3:w267) -> (0:w264:i32)  [unwired: 1 out]
                n160 = property on="Test Ring" class="Ring (strict)"("Value"=w264, "Strings []"=w263) -> ()  [unwired: 2 in, 2 out]
                n161 = property on="Test Ring" class="Ring (strict)"("Visible"=TRUE) -> ()  [unwired: 2 in, 2 out]
                n162 = property on="Test Slider" class="Slide (strict)"("Visible"=FALSE) -> ()  [unwired: 2 in, 2 out]
              }
              frame "White Balance  **" {
                n163 = Index Array(array=w274, index=1) -> (element=w275:cluster{string[]})
                n164 = call <vilib>:"NT Read String.vi"("name"=w277) -> ("value"=w276:string)  [unwired: 8 in, 2 out]
                n165 = Unbundle(w275) -> (w272:string[])
                n166 = Match First String(2:w272, 3:w276) -> (0:w271:i32)  [unwired: 1 out]
                n167 = property on="Test Ring" class="Ring (strict)"("Value"=w271, "Strings []"=w272) -> ()  [unwired: 2 in, 2 out]
                n168 = property on="Test Ring" class="Ring (strict)"("Visible"=TRUE) -> ()  [unwired: 2 in, 2 out]
                n169 = property on="Test Slider" class="Slide (strict)"("Visible"=FALSE) -> ()  [unwired: 2 in, 2 out]
              }
              frame "Exposure  **" {
                n170 = Index Array(array=w283, index=2) -> (element=w284:cluster{string[]})
                n171 = call <vilib>:"NT Read String.vi"("name"=w286) -> ("value"=w285:string)  [unwired: 8 in, 2 out]
                n172 = Unbundle(w284) -> (w280:string[])
                n173 = Match First String(2:w280, 3:w285) -> (0:w281:i32)  [unwired: 1 out]
                n174 = property on="Test Ring" class="Ring (strict)"("Value"=w281, "Strings []"=w280) -> ()  [unwired: 2 in, 2 out]
                n175 = property on="Test Ring" class="Ring (strict)"("Visible"=TRUE) -> ()  [unwired: 2 in, 2 out]
                n176 = property on="Test Slider" class="Slide (strict)"("Visible"=FALSE) -> ()  [unwired: 2 in, 2 out]
              }
              frame "Exposure Priority  **" {
                n177 = Index Array(array=w292, index=3) -> (element=w293:cluster{string[]})
                n178 = call <vilib>:"NT Read String.vi"("name"=w295) -> ("value"=w294:string)  [unwired: 8 in, 2 out]
                n179 = Unbundle(w293) -> (w289:string[])
                n180 = Match First String(2:w289, 3:w294) -> (0:w290:i32)  [unwired: 1 out]
                n181 = property on="Test Ring" class="Ring (strict)"("Value"=w290, "Strings []"=w289) -> ()  [unwired: 2 in, 2 out]
                n182 = property on="Test Ring" class="Ring (strict)"("Visible"=TRUE) -> ()  [unwired: 2 in, 2 out]
                n183 = property on="Test Slider" class="Slide (strict)"("Visible"=FALSE) -> ()  [unwired: 2 in, 2 out]
              }
              frame "Color Enable  **" {
                n184 = Index Array(array=w301, index=4) -> (element=w302:cluster{string[]})
                n185 = call <vilib>:"NT Read String.vi"("name"=w304) -> ("value"=w303:string)  [unwired: 8 in, 2 out]
                n186 = Unbundle(w302) -> (w298:string[])
                n187 = Match First String(2:w298, 3:w303) -> (0:w299:i32)  [unwired: 1 out]
                n188 = property on="Test Ring" class="Ring (strict)"("Value"=w299, "Strings []"=w298) -> ()  [unwired: 2 in, 2 out]
                n189 = property on="Test Ring" class="Ring (strict)"("Visible"=TRUE) -> ()  [unwired: 2 in, 2 out]
                n190 = property on="Test Slider" class="Slide (strict)"("Visible"=FALSE) -> ()  [unwired: 2 in, 2 out]
              }
              frame Default {
                n191 = property on="Test Ring" class="Ring (strict)"("Visible"=FALSE) -> ()  [unwired: 2 in, 2 out]
                n192 = property on="Test Slider" class="Slide (strict)"("Visible"=FALSE) -> ()  [unwired: 2 in, 2 out]
              }
              frame "Brightness  **", "Color Level  **", "Compression  **", "FPS  **", "Sharpness  **" {
                n193 = call <vilib>:"NT Read Number.vi"("name"=w310) -> ("value"=w309:dbl)  [unwired: 8 in, 2 out]
                n194 = local write "Test Slider"(w309) -> ()
                n195 = property on="Test Slider" class="Slide (strict)"("Visible"=TRUE, "Scale.Maximum"=100.0 ("Scale.Range:Maximum")) -> ()  [unwired: 2 in, 2 out]
                n196 = property on="Test Ring" class="Ring (strict)"("Visible"=FALSE) -> ()  [unwired: 2 in, 2 out]
              }
            }
          }
        }
        n197 = property on="Progress" class="Clust (strict)"("Visible"=FALSE) -> ()  [unwired: 2 in, 2 out]
      }
      event "Test Name": Mouse Enter {
        # "Populate the ring with the list of tests"
        n198 = event-data() -> ()  [unwired: 1 in, 1 out]
        n199 = call <vilib>:"NT Read String Array.vi"("name"="TestMode/TestList" ("Name")) -> ("value"=w317:string[])  [unwired: 8 in, 2 out]
        n200 = Build Array (concatenate)("Select the test to run...", w317) -> (w316:string[])
        n201 = property on="Test Name" class="Ring (strict)"("Strings []"=w316) -> ()  [unwired: 2 in, 2 out]
      }
      event "Test Name": Value Change {
        w318 = FALSE ("Visible")
        # "Tell the robot the test name to run"
        n202 = event-data() -> ("NewVal"=w322:u16)  [unwired: 1 in]
        n203 = property on="Test Name" class="Ring (strict)"() -> ("Strings []"=w323:string[])  [unwired: 2 in, 2 out]
        n204 = local write "Progress"(T6 {"Test Progress"=0, "Test Progress Text"=""} ("Progress")) -> ()
        n205 = Index Array(array=w323, index=w322) -> (element=w321:string)
        n206 = call <vilib>:"NT Write String.vi"("value"=w321, "name"="TestMode/TestName" ("Name")) -> ()  [unwired: 9 in, 1 out]
        n207 = property on="Progress" class="Clust (strict)"("Visible"=TRUE) -> ()  [unwired: 2 in, 2 out]
        n208 = property on="Motor" class="Clust (strict)"("Visible"=w318) -> ()  [unwired: 2 in, 2 out]
        n209 = property on="Test Slider" class="Slide (strict)"("Visible"=w318) -> ()  [unwired: 2 in, 2 out]
        n210 = property on="On/Off" class="Bool (strict)"("Visible"=w318) -> ()  [unwired: 2 in, 2 out]
        n211 = property on="Rev/Fwd" class="Clust (strict)"("Visible"=w318) -> ()  [unwired: 2 in, 2 out]
        n212 = property on="Test Ring" class="Ring (strict)"("Visible"=w318) -> ()  [unwired: 2 in, 2 out]
      }
      event "Motor.Enable": Value Change {
        # "When the test mode otor enable helper is set, update that\ntree row item's value"
        n213 = event-data() -> ("NewVal"=w329:bool)  [unwired: 1 in]
        n214 = Unbundle("Motor") -> ("Value"=w328:dbl)  [unwired: 1 out]
        n215 = Select(t=w328, s=w329, f=0.0) -> (s? t:f=w326:dbl)
        n216 = call <vilib>:"NT Write Number.vi"("value"=w326, "name"=w325) -> ()  [unwired: 9 in, 1 out]
      }
      event "Test Slider": Value Change {
        # "When the test mode slider helper is set, update that\ntree row item's value"
        n217 = event-data() -> ("NewVal"=w331:dbl)  [unwired: 1 in]
        n218 = call <vilib>:"NT Write Number.vi"("value"=w331, "name"=w332) -> ()  [unwired: 9 in, 1 out]
      }
      event "On/Off": Value Change {
        # "When the test mode on/off helper value is set, update that\ntree row item's value"
        n219 = event-data() -> ("NewVal"=w335:bool)  [unwired: 1 in]
        n220 = Boolean To (0,1)(Boolean=w335) -> (0, 1=w334:i16)
        n221 = call <vilib>:"NT Write Number.vi"("value"=w334, "name"=w333) -> ()  [unwired: 9 in, 1 out]
      }
      event "Rev/Fwd": Value Change {
        # "When the test mode helper value for relays is set, update that\ntree row item's value"
        n222 = event-data() -> ("NewVal.Forward"=w342:bool, "NewVal.Reverse"=w341:bool)  [unwired: 1 in]
        n223 = Boolean To (0,1)(Boolean=w342) -> (0, 1=w338:i16)
        n224 = Boolean To (0,1)(Boolean=w341) -> (0, 1=w340:i16)
        n225 = Negate(x=w340) -> (-x=w339:i16)
        n226 = Add(x=w338, y=w339) -> (x+y=w337:i16)
        n227 = call <vilib>:"NT Write Number.vi"("value"=w337, "name"=w336) -> ()  [unwired: 9 in, 1 out]
      }
      event "Test Ring": Value Change {
        # "When a test mode helper value is selected from the ring,\nset the tree item's variable to the string value"
        n228 = event-data() -> ("NewVal"=w345:u16)  [unwired: 1 in]
        n229 = property on="Test Ring" class="Ring (strict)"() -> ("Strings []"=w346:string[])  [unwired: 2 in, 2 out]
        n230 = Index Array(array=w346, index=w345) -> (element=w344:string)
        n231 = call <vilib>:"NT Write String.vi"("value"=w344, "name"=w343) -> ()  [unwired: 9 in, 1 out]
      }
      event "Rec Mode": Value Change {
        # "Update globals for recording mode and path to read log from.\nClear when logging and let NetworkTables set path for vision to\nuse."
        n232 = event-data() -> ("NewVal"=w355:enum32{"Stop", "Record", "Playback"})  [unwired: 1 in]
        n233 = global write "WPI_DashboardLogging Global.vi" "Logging Filename"(path "") -> ()
        n234 = global write "WPI_DashboardLogging Global.vi" "Recording"(w355) -> ()
        n235 = case shown="\"Playback\"" w355 {
          tunnel: w354 -> [_ w357 w365]
          tunnel: [_ _ w364] -> w352
          tunnel: [_ _ w363] -> _
          tunnel: w350 -> [_ _ w361]
          tunnel: cluster{i32, i32} {-250, 170} -> [_ _ w360]
          tunnel: [_ _ T24 {"Image Size"=TRUE, "Image Type"=TRUE, "Pixel Value"=TRUE, "ROI Information"=TRUE, "Zoom Factor"=FALSE} ("Image Information Shown:All Elements")] -> w347
          tunnel: [_ _ TRUE ("Zoom Factor")] -> w348
          frame Default {
          }
          frame "Stop", "Record" {
            # "Place Window too"
            n236 = invoke class="VI" method="FP.Close"(reference=w357) -> (reference out=w356:refnum<vi>)  [unwired: 2 in, 2 out]
            n237 = invoke class="VI" method="Abort VI"(reference=w356) -> ()  [unwired: 2 in, 3 out]
          }
          frame "Playback" {
            n238 = call "Open Playback Panel.vi"("Offset"=w360, "DB VI Ref"=w361, "Playback in"=w365) -> ("Playback out"=w362:refnum<vi>)  [unwired: 8 in]
            n239 = register-events(w362) -> (reference out=w364:refnum<event-registration>, error out=w363:errorcluster)  [unwired: 2 in]
          }
        }
        n240 = property on="Camera Image Right" class="ImageControl"("Image Information Shown"=w347, "Image Information Visible"=w348) -> ()  [unwired: 2 in, 2 out]
        n241 = property on="Camera Image" class="ImageControl"("Image Information Shown"=w347, "Image Information Visible"=w348) -> ()  [unwired: 2 in, 2 out]
        n242 = call <vilib>:"WPI_DashboardNT Log FieldName Cache.vi"("Operation"=enum16{"Lookup/Add", "Index", "Clear"}."Clear") -> ()  [unwired: 8 in, 3 out]
      }
      event Panel Close {
        w366 = enum32{"Stop", "Record", "Playback"}."Stop" ("Rec Mode")
        # "Playback window has been closed, abort"
        n243 = event-data() -> ()  [unwired: 1 in, 4 out]
        n244 = local write "Rec Mode"(w366) -> ()
        n245 = global write "WPI_DashboardLogging Global.vi" "Recording"(w366) -> ()
      }
      event Panel Close {
        # "Abort playback window and ourself"
        n246 = event-data() -> ()  [unwired: 1 in, 4 out]
        n247 = invoke class="VI" method="FP.Close"(reference=w369) -> (reference out=w368:refnum<vi>)  [unwired: 2 in, 2 out]
        n248 = invoke class="VI" method="Abort VI"(reference=w368) -> (error out=w367:errorcluster)  [unwired: 2 in, 2 out]
        n249 = invoke class="VI" method="Abort VI"(error in=w367) -> ()  [unwired: 2 in, 3 out]
      }
      event "Tree": Double Click {
        n250 = event-data() -> ("PlatMods"=w375:T26, "Tag"=w372:string)  [unwired: 1 in]
        n251 = Unbundle(w375) -> ("Shift"=w374:bool)  [unwired: 4 out]
        n252 = String Subset(string=w372, length (rest)=1 ("length (rest)")) -> (substring=w371:string)  [unwired: 1 in]
        n253 = Not(x=w374) -> (.not. x?=w373:bool)
        n254 = case shown="\"/\"" w371 {
          tunnel: w372 -> [_ w377]
          tunnel: w373 -> [_ w376]
          frame Default {
          }
          frame "/" {
            n255 = call <vilib>:"NT Update Persistence.vi"("Persistence"=w376, "Name"=w377) -> ()  [unwired: 9 in, 1 out]
          }
        }
      }
    }
  }
  n256 = while {
    tunnel: w35 -> [w379]
    i -> [w382]
    stop <- FALSE stop-if-true
    n257 = Wait (ms)(milliseconds to wait=u32 100) -> ()  [unwired: 1 out]
    n258 = case shown="\"Playback\"" "Rec Mode" {
      tunnel: w382 -> [_ _ w397]
      tunnel: [u32 2829099 ("Base Color") u32 11141120 ("Target Color") w386] -> w378
      frame "Stop", Default {
        # "Reset the color, extra updates don't cost much"
      }
      frame "Record" {
      }
      frame "Playback" {
        # "Playback"
        n259 = Quotient & Remainder(x=w397, y=u32 50 ("milliseconds to wait")) -> (x-y*floor(x/y)=w393:u32)  [unwired: 1 out]
        n260 = Divide(x=w393, y=u32 50 ("milliseconds to wait")) -> (x/y=w390:dbl)
        n261 = Multiply(x=6.283185307179586, y=w390) -> (x*y=w395:dbl)
        n262 = Sine(x=w395) -> (sin(x)=w394:dbl)
        n263 = Absolute Value(x=w394) -> (abs(x)=w387:dbl)
        n264 = call "Interpolate RGB Color.vi"("Proportion"=w387, "Target Color"=u32 30976, "Base Color"=u32 2829099) -> ("Result Color"=w386:u32)  [unwired: 8 in]
      }
    }
    n265 = property class="Pane"(reference=w379, "PaneColor"=w378) -> ()  [unwired: 1 in, 2 out]
  }
  n266 = property on="RR" class="Bool (strict)"("Position"=w7) -> ()  [unwired: 2 in, 2 out]
  n267 = local write "Dashboard Tab"(T2."Swerve Diagnostics" ("Dashboard Tab")) -> ()
  n268 = property on="On/Off" class="Bool (strict)"("Visible"=w28) -> ()  [unwired: 2 in, 2 out]
  n269 = property on="Motor" class="Clust (strict)"("Visible"=w28) -> ()  [unwired: 2 in, 2 out]
  n270 = property on="Progress" class="Clust (strict)"("Visible"=w28) -> ()  [unwired: 2 in, 2 out]
  n271 = property on="Test Ring" class="Ring (strict)"("Visible"=w28) -> ()  [unwired: 2 in, 2 out]
  n272 = property on="Rev/Fwd" class="Clust (strict)"("Visible"=w28) -> ()  [unwired: 2 in, 2 out]
  n273 = while {
    tunnel: u16 1741 ("timeout ms (25000)") -> [w399]
    stop <- FALSE stop-if-true
    n274 = TCP Create Listener(10:w399) -> (0:w398:errorcluster, 3:w400:refnum<k5>)  [unwired: 4 in, 1 out]
    n275 = case shown="No Error" w398 {
      selector: w398 -> [w402 _]
      tunnel: w400 -> [w403 _]
      frame No Error {
        n276 = while {
          tunnel: w403 -> [w406]
          tunnel: w402 -> [w405]
          stop <- FALSE stop-if-true
          n277 = TCP Wait On Listener(8:w405, 11:w406) -> (0:w407:errorcluster, 4:w408:refnum<k5>)  [unwired: 2 in, 3 out]
          n278 = local write "TCP"(w408) -> ()
          n279 = case shown="Error" w407 {
            frame No Error {
            }
            frame Error {
              n280 = Wait (ms)(milliseconds to wait=u32 1000) -> ()  [unwired: 1 out]
            }
          }
        }
      }
      frame Error {
        n281 = Wait (ms)(milliseconds to wait=u32 1000) -> ()  [unwired: 1 out]
      }
    }
  }
  n282 = global write "WPI_DashboardLogging Global.vi" "Recording"(w30) -> ()
  n283 = local write "Rec Mode"(w30) -> ()
  n284 = call <vilib>:"NT Write String.vi"("name"="Auto Selector" ("Name")) -> ()  [unwired: 10 in, 1 out]
